vi "network stream connection status trial with reconnect.vi"() -> ()   [LabVIEW 2018]
uses:
  <resource>/objmgr/ni.dex.rc
panel:
  out "connection attempts":i32
  out "error out":errorcluster
  out "timed out?":bool
  out "Remote Endpoint Destroyed":bool
  out "Number of Disconnections":u32
  out "Is Connected":bool
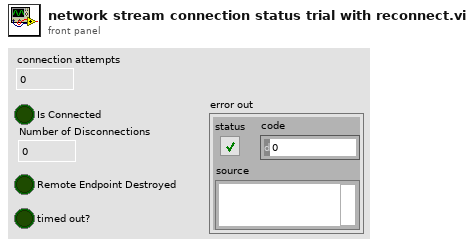
[diagram p1: front panel]
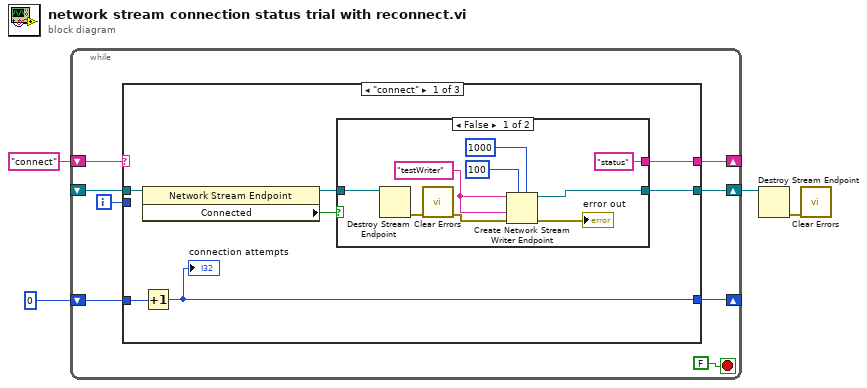
[diagram p0: block diagram]
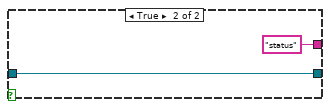
[diagram p2: hidden frame]
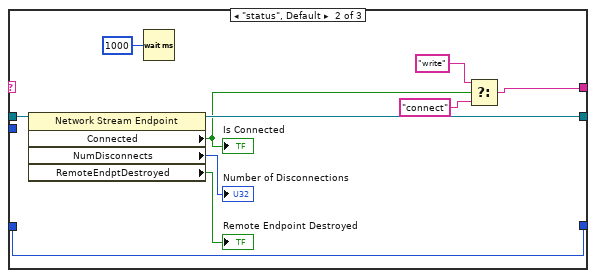
[diagram p3: hidden frame]
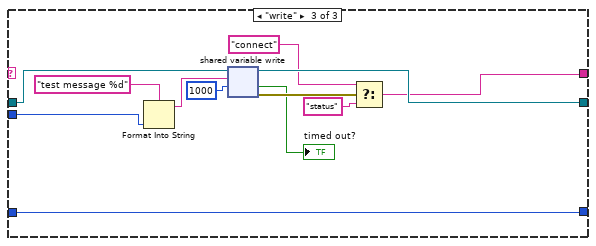
[diagram p4: hidden frame]
diagram:
  n1 = while {
    shift-right: [w10] -> w3
    shift-left: _ -> [w9]
    shift-right: [w8] -> _
    shift-left: "connect" ("writer name") -> [w12]
    shift-right: [w5] -> _
    shift-left: 0 -> [w6]
    i -> [w7]
    stop <- FALSE stop-if-true
    n2 = case shown="\"connect\"" w12 {
      tunnel: [w19 w37 w48] -> w10
      tunnel: w9 -> [w17 w40 w52]
      tunnel: [w18 w33 w44] -> w8
      tunnel: w7 -> [_ _ w51]
      tunnel: w6 -> [w14 w31 w41]
      tunnel: [w13 w31 w41] -> w5
      frame "connect" {
        n3 = property class="Network Stream Endpoint"(reference=w17) -> (reference out=w15:refnum<k21>, "Connected"=w16:bool)  [unwired: 1 in, 1 out]
        n4 = Increment(x=w14) -> (x+1=w13:i32)
        "connection attempts" <- w13
        n5 = case shown="False" w16 {
          tunnel: [w25 w30] -> w19
          tunnel: ["status" ("writer name") "status" ("writer name")] -> w18
          tunnel: w15 -> [w24 w30]
          frame False {
            w28 = "testWriter" ("writer name")
            n6 = Destroy Stream Endpoint(11:w24) -> (0:w23:errorcluster)  [unwired: 1 in]
            n7 = call <vilib>:"Clear Errors.vi"("error in (no error)"=w23) -> ("error out"=w22:errorcluster)  [unwired: 5 in, 1 out]
            n8 = Create Network Stream Writer Endpoint(5:1000 ("timeout in ms (-1)"), 7:100 ("writer buffer size"), 8:w22, 9:w28, 11:w28) -> (0:→"error out":errorcluster, 3:w25:refnum<k21>)  [unwired: 2 in]
          }
          frame True {
          }
        }
      }
      frame "status", Default {
        n9 = property class="Network Stream Endpoint"(reference=w40) -> (reference out=w37:refnum<k21>, "Connected"=w35:bool, "NumDisconnects"=→"Number of Disconnections":u32, "RemoteEndptDestroyed"=→"Remote Endpoint Destroyed":bool)  [unwired: 1 in, 1 out]
        "Is Connected" <- w35
        n10 = Wait (ms)(milliseconds to wait=u32 1000) -> ()  [unwired: 1 out]
        n11 = Select(t="write" ("writer name"), s=w35, f="connect" ("writer name")) -> (s? t:f=w33:string)
      }
      frame "write" {
        n12 = Format Into String(format string="test message %d" ("data in"), w51) -> (resulting string=w49:string)  [unwired: 2 in, 1 out]
        n13 = shared-variable-write(w52, w49, 1000 ("timeout ms (-1)")) -> (w48:refnum<k21>, w43:errorcluster, →"timed out?":bool)  [unwired: 1 in]
        n14 = Select(t="connect" ("writer name"), s=w43, f="status" ("writer name")) -> (s? t:f=w44:string)
      }
    }
  }
  n15 = Destroy Stream Endpoint(11:w3) -> (0:w2:errorcluster)  [unwired: 1 in]
  n16 = call <vilib>:"Clear Errors.vi"("error in (no error)"=w2) -> ()  [unwired: 5 in, 2 out]
